vi "PXIe-4139 Init Channel (RT).vi"(5 "Channel Type":T3 items=["Voltage Controlled", "Current Controlled"], 7 "Channel Sense":T2=1008 items=["Local"=1008, "Remote"=1009], 8 "error in (no error)":errorcluster, 10 "resource name":refnum<k15>="Dev1", 11 "Device Reference In":T1 format="%.0x") -> (0 "error out":errorcluster, 2 "resource name Out":refnum<k15>="Dev1", 3 "Device Reference Out":T1 format="%.0x", 4 "Defaults":dbl[](array[numeric]), 6 "FIFO Indexes":i32[](array[numeric]))   [LabVIEW 2023, in "PXIe-4139 Custom Device.lvlib"]
uses:
  PXIe-4139 Custom Device.lvlib
  Controls/Channel Type.ctl
  Controls/Channel Sense.ctl
  <vilib>/NI VeriStand/Custom Device API/Custom Device Item Ref.ctl
  <instrlib>/niDCPower/nidcpower.llb/niDCPower Output Function.ctl
  PXIe-4139 Global Variable.vi
  <vilib>/NI VeriStand/Custom Device Tools/Custom Device Utility Library/NI VeriStand - Search for Item by Property.vi
  <vilib>/NI VeriStand/Custom Device Tools/Custom Device Utility Library/NI VeriStand - Search for Item by Name.vi
  <vilib>/NI VeriStand/Custom Device API/Custom Device API.lvlib
  <vilib>/NI VeriStand/Custom Device Tools/Custom Device Utility Library/Custom Device Utility Library.lvlib
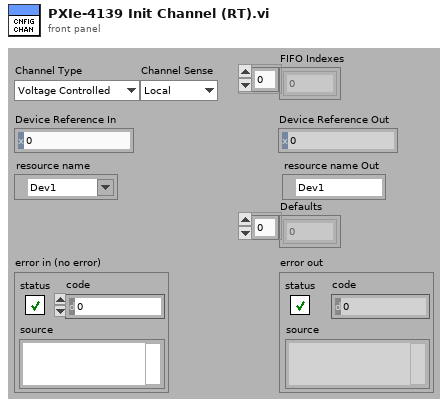
[diagram p1: front panel]
types:
  T1 = typedef "Custom Device API.lvlib/Custom Device Item Ref.ctl" = u64
  T2 = typedef "PXIe-4139 Custom Device.lvlib/Channel Sense.ctl" = i32
  T3 = typedef "PXIe-4139 Custom Device.lvlib/Channel Type.ctl" = i32
  T4 = typedef "Custom Device API.lvlib/Custom Device Channel.ctl" = cluster{"Type":T5, "Units":string, "Default Value":dbl, "Faultable":bool, "Scalable":bool}
  T5 = typedef "Custom Device API.lvlib/Custom Device Channel Type.ctl" = enum16{"Input", "Output"}
  T6 = typedef "niDCPower Output Function.ctl" = i32
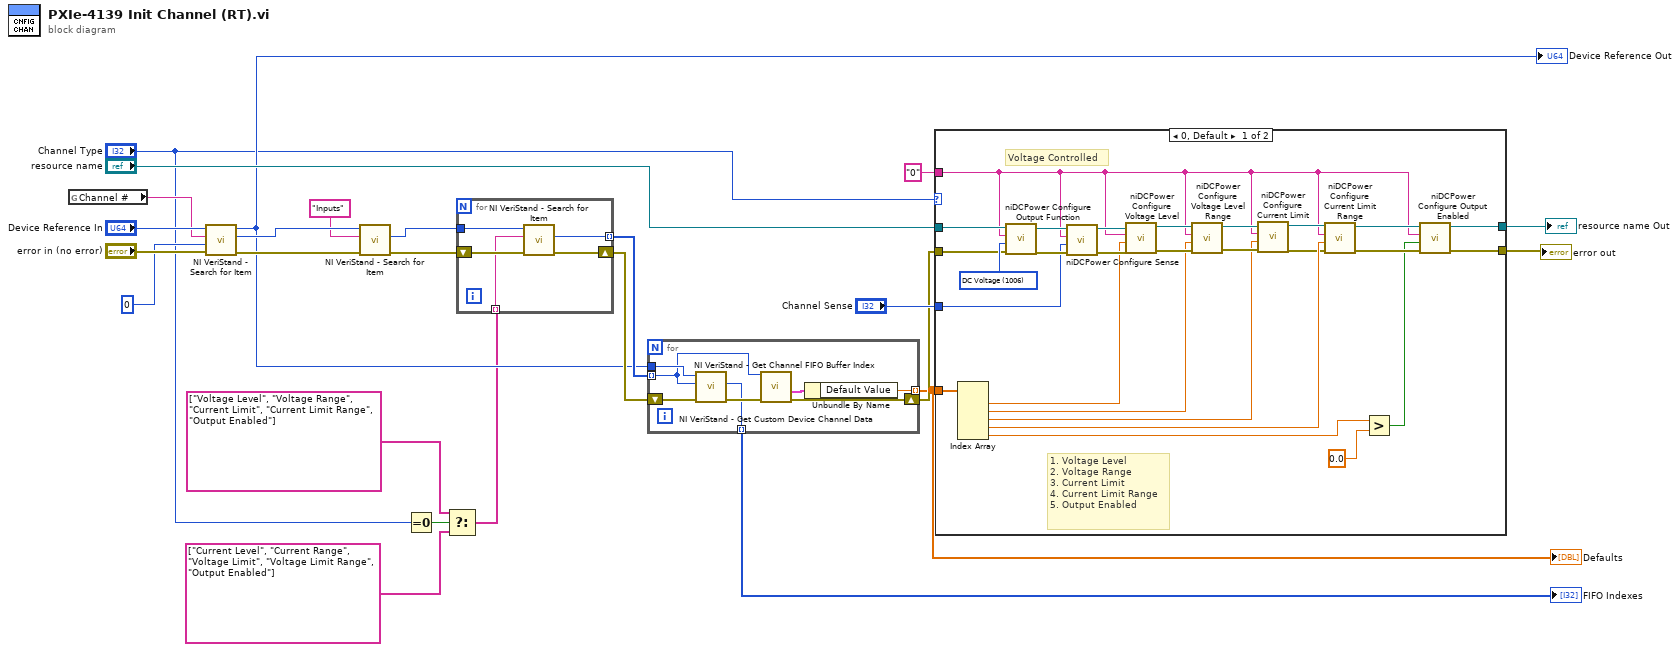
[diagram p0: block diagram]
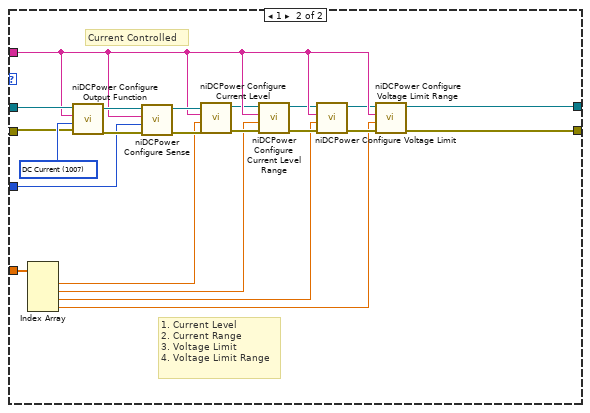
[diagram p2: hidden frame]
diagram:
  n1 = global read "PXIe-4139 Global Variable.vi" "Channel #"() -> (w20:string)
  n2 = call-poly <vilib>:"NI VeriStand - Search for Item.vi"("error in"="error in (no error)", "Property Value"=0, "Property Name"=w20, "Section Ref in"="Device Reference In") -> ("error out"=w21:errorcluster, "Item Ref"=w18:T1, "Section Ref out"=w9:T1)  [unwired: 4 in, 1 out]
  "Device Reference Out" <- w9
  n3 = call-poly <vilib>:"NI VeriStand - Search for Item.vi"("error in"=w21, "Item Name"="Inputs" ("Channel Name"), "Section Ref in"=w18) -> ("error out"=w16:errorcluster, "Item Ref"=w12:T1)  [unwired: 5 in, 2 out]
  n4 = Equal To 0?(x="Channel Type") -> (x = 0?=w4:bool)
  n5 = Select(t=string[] ["Voltage Level", "Voltage Range", "Current Limit", "Current Limit Range", "Output Enabled"], s=w4, f=string[] ["Current Level", "Current Range", "Voltage Limit", "Voltage Limit Range", "Output Enabled"]) -> (s? t:f=w1:string[])
  n6 = for {
    tunnel: w12 -> [w29]
    tunnel: [w27] -> w10 mode=indexing
    shift-right: [w28] -> w11
    shift-left: w16 -> [w30]
    tunnel: w1 -> [w26] mode=indexing
    n7 = call-poly <vilib>:"NI VeriStand - Search for Item.vi"("error in"=w30, "Item Name"=w26, "Section Ref in"=w29) -> ("error out"=w28:errorcluster, "Item Ref"=w27:T1)  [unwired: 5 in, 2 out]
  }
  n8 = for {
    tunnel: w10 -> [w32] mode=indexing
    tunnel: [w37] -> w6 mode=indexing
    shift-right: [w35] -> w8
    shift-left: w11 -> [w36]
    tunnel: w9 -> [w33]
    tunnel: [w31] -> w7 mode=indexing
    n9 = call <vilib>:"NI VeriStand - Get Channel FIFO Buffer Index.vi"("error in"=w36, "Channel Ref"=w32, "Device Ref in"=w33) -> ("error out"=w34:errorcluster, "Channel FIFO Buffer Index"=w31:i32)  [unwired: 4 in, 3 out]
    n10 = call <vilib>:"NI VeriStand - Get Custom Device Channel Data.vi"("error in (no error)"=w34, "Channel Ref in"=w32) -> ("error out"=w35:errorcluster, "Channel"=w38:T4)  [unwired: 4 in, 4 out]
    n11 = Unbundle By Name(w38) -> ("Default Value"=w37:dbl)
  }
  "FIFO Indexes" <- w7
  "Defaults" <- w6
  n12 = case shown="0, Default" "Channel Type" {
    tunnel: w8 -> [w48 w67]
    tunnel: "resource name" -> [w62 w81]
    tunnel: "Channel Sense" -> [w59 w78]
    tunnel: [w43 w83] -> w23
    tunnel: [w42 w82] -> w24
    tunnel: "0" ("Channel Name") -> [w44 w79]
    tunnel: w6 -> [w47 w66]
    frame 0, Default {
      w65 = T6 1006 items=["DC Voltage"=1006, "DC Current"=1007] ("output function")
      # "1. Voltage Level\n2. Voltage Range\n3. Current Limit\n4. Current Limit Range\n5. Output Enabled"
      # "Voltage Controlled"
      n13 = Index Array(array=w47) -> (element #1=w58:dbl, element #2=w50:dbl, element #3=w49:dbl, element #4=w57:dbl, element #5=w41:dbl)  [unwired: 5 in]
      n14 = call <instrlib>:"niDCPower Configure Output Function.vi"("error in (no error)"=w48, "output function"=w65, "channel name"=w44, "instrument handle"=w62) -> ("error out"=w63:errorcluster, "instrument handle out"=w64:refnum<k15>)  [unwired: 6 in]
      n15 = call <instrlib>:"niDCPower Configure Sense.vi"("error in (no error)"=w63, "sense"=w59, "channel name"=w44, "instrument handle"=w64) -> ("error out"=w61:errorcluster, "instrument handle out"=w60:refnum<k15>)  [unwired: 6 in]
      n16 = call <instrlib>:"niDCPower Configure Voltage Level.vi"("error in (no error)"=w61, "voltage level"=w58, "channel name"=w44, "instrument handle"=w60) -> ("error out"=w51:errorcluster, "instrument handle out"=w56:refnum<k15>)  [unwired: 6 in]
      n17 = call <instrlib>:"niDCPower Configure Voltage Level Range.vi"("error in (no error)"=w51, "voltage level range"=w50, "channel name"=w44, "instrument handle"=w56) -> ("error out"=w52:errorcluster, "instrument handle out"=w55:refnum<k15>)  [unwired: 6 in]
      n18 = call <instrlib>:"niDCPower Configure Current Limit.vi"("error in (no error)"=w52, "current limit"=w49, "channel name"=w44, "instrument handle"=w55) -> ("error out"=w53:errorcluster, "instrument handle out"=w54:refnum<k15>)  [unwired: 6 in]
      n19 = call <instrlib>:"niDCPower Configure Current Limit Range.vi"("error in (no error)"=w53, "current limit range"=w57, "channel name"=w44, "instrument handle"=w54) -> ("error out"=w45:errorcluster, "instrument handle out"=w46:refnum<k15>)  [unwired: 6 in]
      n20 = Greater?(x=w41, y=0.0) -> (0:w39:bool)
      n21 = call <instrlib>:"niDCPower Configure Output Enabled.vi"("error in (no error)"=w45, "output enabled"=w39, "channel name"=w44, "instrument handle"=w46) -> ("error out"=w42:errorcluster, "instrument handle out"=w43:refnum<k15>)  [unwired: 6 in]
    }
    frame 1 {
      w80 = T6 1007 items=["DC Voltage"=1006, "DC Current"=1007] ("output function")
      # "1. Current Level\n2. Current Range\n3. Voltage Limit\n4. Voltage Limit Range"
      # "Current Controlled"
      n22 = Index Array(array=w66) -> (element #1=w71:dbl, element #2=w70:dbl, element #3=w69:dbl, element #4=w68:dbl)  [unwired: 4 in]
      n23 = call <instrlib>:"niDCPower Configure Output Function.vi"("error in (no error)"=w67, "output function"=w80, "channel name"=w79, "instrument handle"=w81) -> ("error out"=w85:errorcluster, "instrument handle out"=w84:refnum<k15>)  [unwired: 6 in]
      n24 = call <instrlib>:"niDCPower Configure Sense.vi"("error in (no error)"=w85, "sense"=w78, "channel name"=w79, "instrument handle"=w84) -> ("error out"=w86:errorcluster, "instrument handle out"=w87:refnum<k15>)  [unwired: 6 in]
      n25 = call <instrlib>:"niDCPower Configure Current Level.vi"("error in (no error)"=w86, "current level"=w71, "channel name"=w79, "instrument handle"=w87) -> ("error out"=w72:errorcluster, "instrument handle out"=w73:refnum<k15>)  [unwired: 6 in]
      n26 = call <instrlib>:"niDCPower Configure Current Level Range.vi"("error in (no error)"=w72, "current level range"=w70, "channel name"=w79, "instrument handle"=w73) -> ("error out"=w74:errorcluster, "instrument handle out"=w77:refnum<k15>)  [unwired: 6 in]
      n27 = call <instrlib>:"niDCPower Configure Voltage Limit.vi"("error in (no error)"=w74, "voltage limit"=w69, "channel name"=w79, "instrument handle"=w77) -> ("error out"=w75:errorcluster, "instrument handle out"=w76:refnum<k15>)  [unwired: 6 in]
      n28 = call <instrlib>:"niDCPower Configure Voltage Limit Range.vi"("error in (no error)"=w75, "voltage limit range"=w68, "channel name"=w79, "instrument handle"=w76) -> ("error out"=w82:errorcluster, "instrument handle out"=w83:refnum<k15>)  [unwired: 6 in]
    }
  }
  "error out" <- w24
  "resource name Out" <- w23
